vi "ImagingAnalyzer.vi"() -> ()   [LabVIEW 2012]
uses:
  <instrlib>/niScope/Controls/niScope trigger source.ctl
  <instrlib>/niScope/Controls/niScope vertical coupling.ctl
  <instrlib>/niScope/Configure/Trigger/niScope Configure Trigger Edge.vi
  <instrlib>/niScope/Acquire/Fetch/niScope Multi Fetch Cluster.vi
panel:
  out "x/y":dbl
  in  "Signal Coupling":T1=1 caption="vertical coupling" items=["AC", "DC", "Ground"]
  in  "Signal Source":T2="1"
  in  "Reference Position (%)":dbl=10.0 caption="Reference Position" format="%.1f"
  out "Total Acquisition Time (us)":dbl
  out "Scope Traces":dbl[](graph)
  in  "min sample rate":dbl=20000000.0 caption="Sample Rate (Max 20M)" format="%^.2e"
  in  "Trigger Level":dbl=2.0 format="%.2f"
  in  "Trigger Source":T2="0"
  in  "Number of Records":i32=1500 caption="Number of Samples"
  # "Settings can be modified \nin real-time (every 10s or so)."
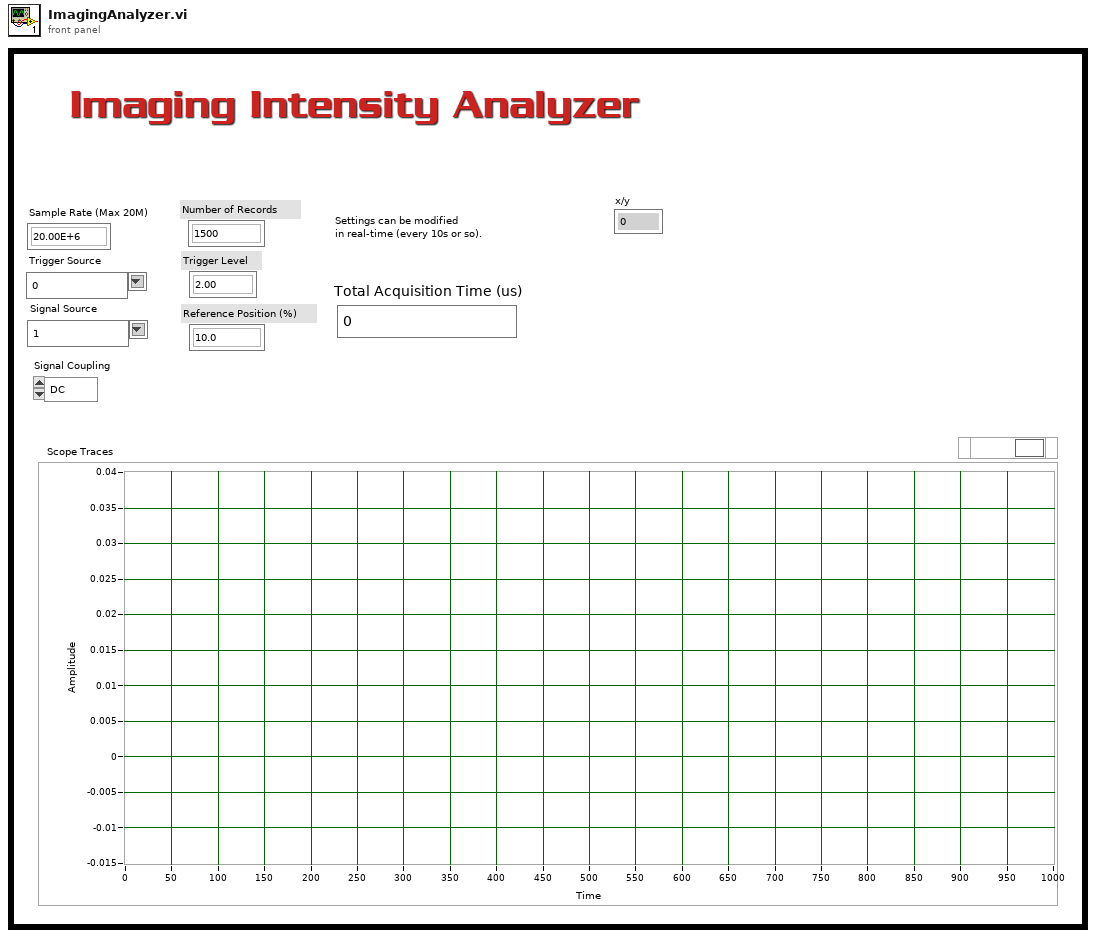
[diagram p1: front panel]
types:
  T1 = typedef "niScope vertical coupling.ctl" = i32
  T2 = typedef "niScope trigger source.ctl" = string
  T3 = cluster{"relativeInitialX":dbl, "xIncrement":dbl, "wfm":dbl[]}[]
  T4 = cluster{"relativeInitialX":dbl, "xIncrement":dbl, "wfm":dbl[]}
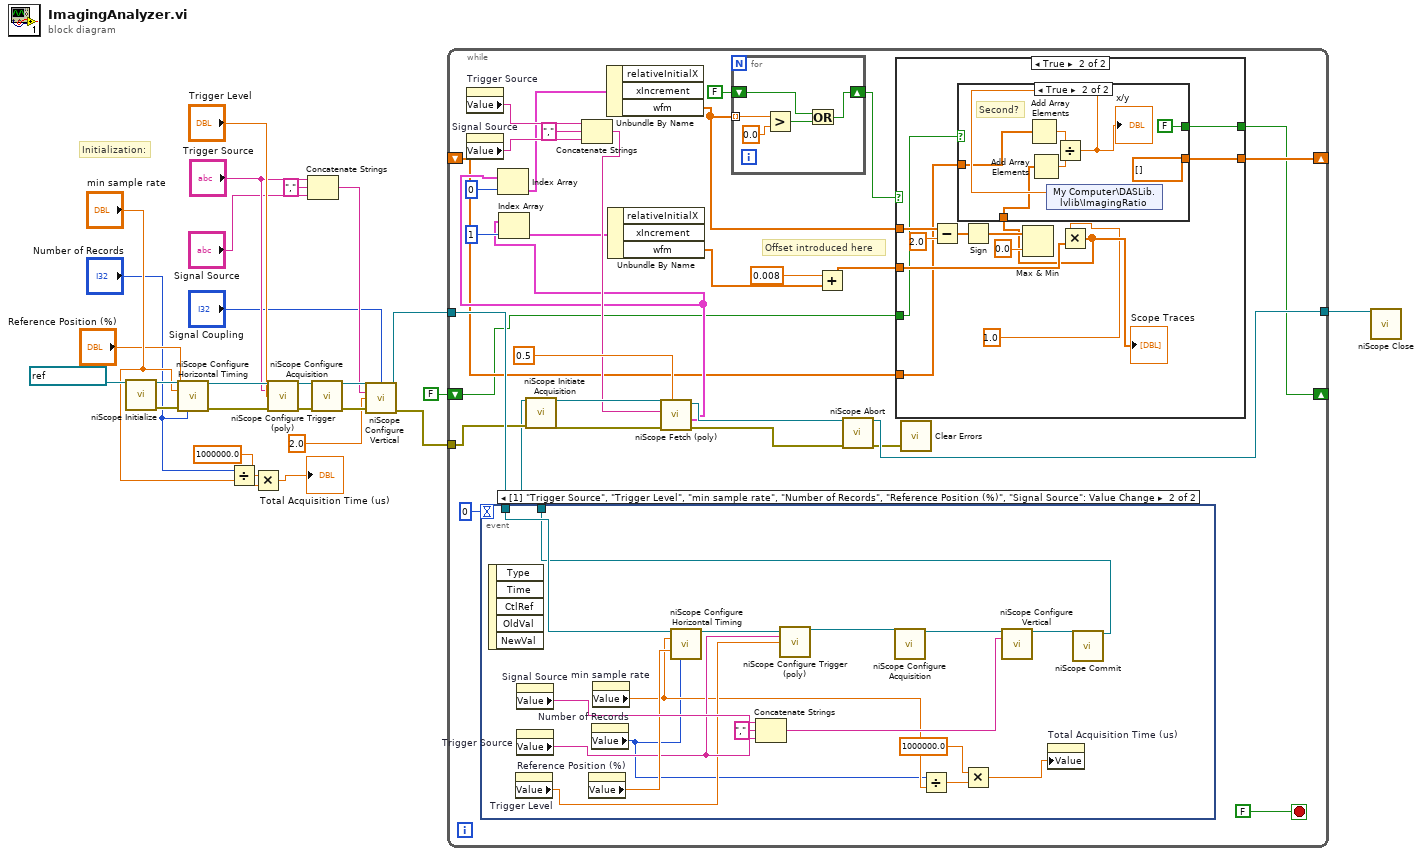
[diagram p0: block diagram]
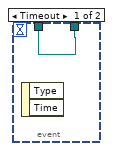
[diagram p2: hidden frame]
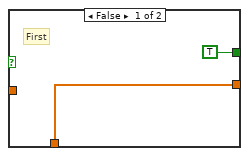
[diagram p4: hidden frame]
diagram:
  # "Initialization:"
  n1 = call <instrlib>:"niScope Initialize.vi"("resource name"=refnum<k15> "PXI1Slot4") -> ("instrument handle"=w25:refnum<k15>, "error out"=w24:errorcluster)  [unwired: 13 in]
  n2 = call <instrlib>:"niScope Configure Horizontal Timing.vi"("instrument handle"=w25, "min sample rate"="min sample rate", "reference position"="Reference Position (%)", "error in"=w24, "min record length"="Number of Records") -> ("instrument handle out"=w23:refnum<k15>, "error out"=w14:errorcluster)  [unwired: 9 in]
  n3 = Divide(x="Number of Records", y="min sample rate") -> (x/y=w12:dbl)
  n4 = Multiply(x=w12, y=1000000.0) -> (x*y=→"Total Acquisition Time (us)":dbl)
  n5 = call-poly <instrlib>:"niScope Configure Trigger (poly).vi"("instrument handle"=w23, "trigger source"="Trigger Source", "trigger level"="Trigger Level", "error in"=w14) -> ("instrument handle out"=w20:refnum<k15>, "error out"=w19:errorcluster)  [unwired: 10 in]
  n6 = Concatenate Strings("Trigger Source", "," ("string"), "Signal Source") -> (w7:string)
  n7 = call <instrlib>:"niScope Configure Acquisition.vi"("instrument handle"=w20, "error in"=w19) -> ("instrument handle out"=w17:refnum<k15>, "error out"=w18:errorcluster)  [unwired: 12 in]
  n8 = call <instrlib>:"niScope Configure Vertical.vi"("instrument handle"=w17, "vertical coupling"="Signal Coupling", "channels"=w7, "vertical range"=2.0, "error in"=w18) -> ("instrument handle out"=w21:refnum<k15>, "error out"=w16:errorcluster)  [unwired: 9 in]
  n9 = while {
    tunnel: w21 -> [w48]
    tunnel: w16 -> [w47]
    tunnel: [w56] -> w15
    shift-right: [w33] -> _
    shift-left: _ -> [w32]
    shift-right: [w31] -> _
    shift-left: FALSE -> [w30]
    stop <- FALSE ("stop") stop-if-true
    # "Offset introduced here"
    n10 = property on="Trigger Source" class="CmbBox (strict)"() -> ("Value"=w44:T2)  [unwired: 2 in, 2 out]
    n11 = property on="Signal Source" class="CmbBox (strict)"() -> ("Value"=w42:T2)  [unwired: 2 in, 2 out]
    n12 = event shown="[1] \"Trigger Source\", \"Trigger Level\", \"min sample rate\", \"Number of Records\", \"Reference Position (%)\", \"Signal Source\": Value Change" {
      selector: _ -> [_ _]
      dyn-events: _ -> [_ _]
      timeout: 0 -> [_ _]
      tunnel: w48 -> [w58 w75]
      tunnel: [w58 w62] -> w34
      event Timeout {
        n13 = event-data() -> ()  [unwired: 1 in, 2 out]
      }
      event "Trigger Level", "min sample rate", "Number of Records", "Reference Position (%)": Value Change {
        n14 = event-data() -> ()  [unwired: 1 in, 5 out]
        n15 = property on="Trigger Level" class="DigNum (strict)"() -> ("Value"=w66:dbl)  [unwired: 2 in, 2 out]
        n16 = property on="Signal Source" class="CmbBox (strict)"() -> ("Value"=w69:T2)  [unwired: 2 in, 2 out]
        n17 = property on="Trigger Source" class="CmbBox (strict)"() -> ("Value"=w67:T2)  [unwired: 2 in, 2 out]
        n18 = property on="Reference Position (%)" class="DigNum (strict)"() -> ("Value"=w68:dbl)  [unwired: 2 in, 2 out]
        n19 = property on="Number of Records" class="DigNum (strict)"() -> ("Value"=w61:i32)  [unwired: 2 in, 2 out]
        n20 = property on="min sample rate" class="DigNum (strict)"() -> ("Value"=w65:dbl)  [unwired: 2 in, 2 out]
        n21 = call <instrlib>:"niScope Configure Horizontal Timing.vi"("instrument handle"=w75, "min sample rate"=w65, "reference position"=w68, "min record length"=w61) -> ("instrument handle out"=w74:refnum<k15>)  [unwired: 10 in, 1 out]
        n22 = Concatenate Strings(w69, "," ("string"), w67) -> (w71:string)
        n23 = call-poly <instrlib>:"niScope Configure Trigger (poly).vi"("instrument handle"=w74, "trigger source"=w67, "trigger level"=w66) -> ("instrument handle out"=w73:refnum<k15>)  [unwired: 11 in, 1 out]
        n24 = call <instrlib>:"niScope Configure Acquisition.vi"("instrument handle"=w73) -> ("instrument handle out"=w72:refnum<k15>)  [unwired: 13 in, 1 out]
        n25 = Divide(x=w61, y=w65) -> (x/y=w64:dbl)
        n26 = Multiply(x=1000000.0 ("y"), y=w64) -> (x*y=w60:dbl)
        n27 = call <instrlib>:"niScope Configure Vertical.vi"("instrument handle"=w72, "channels"=w71) -> ("instrument handle out"=w63:refnum<k15>)  [unwired: 12 in, 1 out]
        n28 = property on="Total Acquisition Time (us)" class="DigNum (strict)"("Value"=w60) -> ()  [unwired: 2 in, 2 out]
        n29 = call <instrlib>:"niScope Commit.vi"("instrument handle"=w63) -> ("instrument handle out"=w62:refnum<k15>)  [unwired: 13 in, 1 out]
      }
    }
    n30 = call <instrlib>:"niScope Initiate Acquisition.vi"("instrument handle"=w34, "error in"=w47) -> ("instrument handle out"=w46:refnum<k15>, "error out"=w40:errorcluster)  [unwired: 12 in]
    n31 = Concatenate Strings(w44, "," ("string"), w42) -> (w41:string)
    n32 = call-poly <instrlib>:"niScope Fetch (poly).vi"("timeout"=0.5, "error in"=w40, "channels"=w41, "instrument handle"=w46) -> ("error out"=w39:errorcluster, "waveform"=w37:T3, "instrument handle out"=w38:refnum<k15>)  [unwired: 4 in, 1 out]
    n33 = Index Array(array=w37, index=0) -> (element=w36:T4)
    n34 = Index Array(array=w37, index=1) -> (element=w35:T4)
    n35 = Unbundle By Name(w36) -> ("wfm"=w29:dbl[])  [unwired: 2 out]
    n36 = Unbundle By Name(w35) -> ("wfm"=w50:dbl[])  [unwired: 2 out]
    n37 = for {
      tunnel: w29 -> [w76] mode=indexing
      shift-right: [w77] -> w52
      shift-left: FALSE -> [w78]
      n38 = Greater?(x=w76, y=0.0) -> (0:w79:bool)
      n39 = Or(x=w78, y=w79) -> (x .or. y?=w77:bool)
    }
    n40 = Add(x=0.008 ("timeout"), y=w50) -> (x+y=w28:dbl[])
    n41 = call <instrlib>:"niScope Abort.vi"("instrument handle"=w38, "error in"=w39) -> ("instrument handle out"=w56:refnum<k15>, "error out"=w55:errorcluster)  [unwired: 12 in]
    n42 = case shown="True" w52 {
      tunnel: w29 -> [_ w90]
      tunnel: w28 -> [_ w89]
      tunnel: [w82 w87] -> w33
      tunnel: w32 -> [w82 w86]
      tunnel: [w81 w85] -> w31
      tunnel: w30 -> [w81 w84]
      frame False {
      }
      frame True {
        n43 = Subtract(x=w90, y=2.0 ("timeout")) -> (x-y=w93:dbl[])
        n44 = Sign(1:w93) -> (0:w92:dbl[])
        n45 = Max & Min(x=w92, y=0.0 ("timeout")) -> ()  [unwired: 2 out]
        n46 = Multiply(x=1.0 ("timeout"), y=w89) -> (x*y=w88:dbl[])
        "Scope Traces" <- w88
        n47 = case shown="True" w84 {
          tunnel: w88 -> [w96 w97]
          tunnel: [w96 dbl[] []] -> w87
          tunnel: w86 -> [_ w98]
          tunnel: [TRUE FALSE] -> w85
          frame False {
            # "First"
          }
          frame True {
            # "Second?"
            n48 = Add Array Elements(numeric array=w98) -> (sum=w101:dbl)
            n49 = Add Array Elements(numeric array=w97) -> (sum=w100:dbl)
            n50 = Divide(x=w101, y=w100) -> (x/y=w99:dbl)
            "x/y" <- w99
            n51 = shared-variable "My Computer\\DASLib.lvlib\\ImagingRatio"(w99) -> ()  [unwired: 1 in, 1 out]
          }
        }
      }
    }
    n52 = call <vilib>:"Clear Errors.vi"("error in (no error)"=w55) -> ()  [unwired: 6 in, 1 out]
  }
  n53 = call <instrlib>:"niScope Close.vi"("instrument handle"=w15) -> ()  [unwired: 14 in, 1 out]
